vi "Tag Names.vi"(11 "Process Name":string) -> (2 "Flow Tags":T1, 4 "All Boolean Tags":string[](array[string]), 5 "All  Numeric Tags":string[](array[string]))   [LabVIEW 2018, in "Flow Module.lvlib" / "Flow Module Engine.lvlib"]
uses:
  Flow Module Engine.lvlib
  Bronkhorst M14 Flow Meter/Tag Cluster.ctl
  Flow Module.lvlib
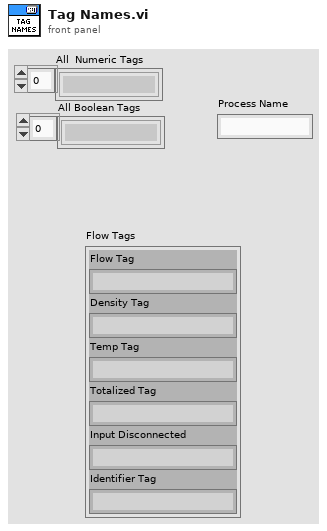
[diagram p1: front panel]
types:
  T1 = typedef "Flow Module.lvlib/Tag Cluster.ctl" = cluster{"Flow Tag":string, "Density Tag":string, "Temp Tag":string, "Totalized Tag":string, "Input Disconnected":string, "Identifier Tag":string}
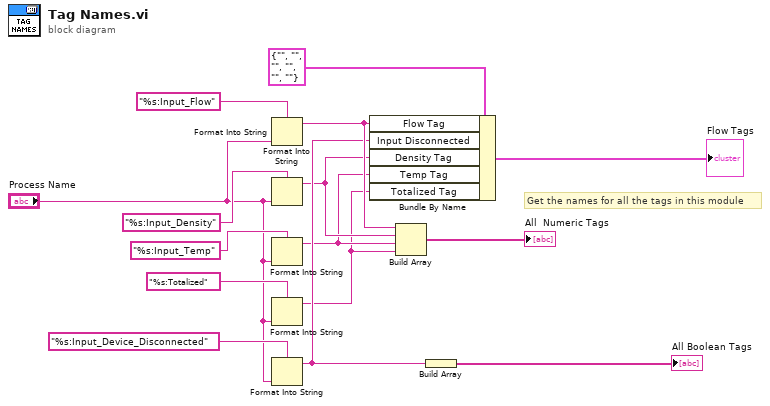
[diagram p0: block diagram]
diagram:
  # "Get the names for all the tags in this module"
  n1 = Format Into String(format string="%s:Input_Flow", "Process Name") -> (resulting string=w11:string)  [unwired: 2 in, 1 out]
  n2 = Format Into String(format string="%s:Input_Density", "Process Name") -> (resulting string=w7:string)  [unwired: 2 in, 1 out]
  n3 = Format Into String(format string="%s:Input_Temp", "Process Name") -> (resulting string=w4:string)  [unwired: 2 in, 1 out]
  n4 = Format Into String(format string="%s:Totalized", "Process Name") -> (resulting string=w1:string)  [unwired: 2 in, 1 out]
  n5 = Format Into String(format string="%s:Input_Device_Disconnected", "Process Name") -> (resulting string=w10:string)  [unwired: 2 in, 1 out]
  n6 = Bundle By Name(cluster=T1 {"Flow Tag"="", "Density Tag"="", "Temp Tag"="", "Totalized Tag"="", "Input Disconnected"="", "Identifier Tag"=""} ("Flow Tags 2"), "Flow Tag"=w11, "Input Disconnected"=w10, "Density Tag"=w7, "Temp Tag"=w4, "Totalized Tag"=w1) -> (→"Flow Tags":T1)
  n7 = Build Array(w11, w7, w4, w1) -> (→"All  Numeric Tags":string[])
  n8 = Build Array(w10) -> (→"All Boolean Tags":string[])
